vi "GETRequest.vi"(6 "Query parameters":cluster{"key":string, "value":string}[](array[cluster]), 8 "error in (no error)":errorcluster, 9 "Parameter":string, 10 "Request":string, 11 "ByteRESTBase in":refnum<class "RESTBase.lvclass">) -> (0 "error out":errorcluster, 1 "Headers":string, 2 "Body":string, 3 "ByteRESTBase out":refnum<class "RESTBase.lvclass">)   [LabVIEW 2019, in "ByteREST.lvlib" / "RESTBase.lvclass"]
doc: "Effettua una richiesta di GET al server come:\nSERVER/api/bytegs/RICHIESTA/PARAMETRO(opzionale)"
uses:
  RESTBase.lvclass
  Status_Code.ctl
  RESTBase.lvclass/RESTBase.ctl
  <vilib>/httpClient/LabVIEWHTTPClient.lvlib
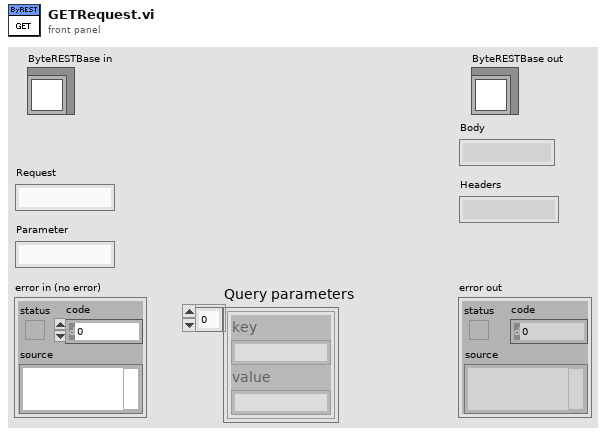
[diagram p1: front panel]
types:
  T1 = typedef "ByteREST.lvlib/RESTBase.lvclass/Status_Code.ctl" = u16
  T2 = typedef "LabVIEWHTTPClient.lvlib/ClientHandle.ctl" = refnum<k1>
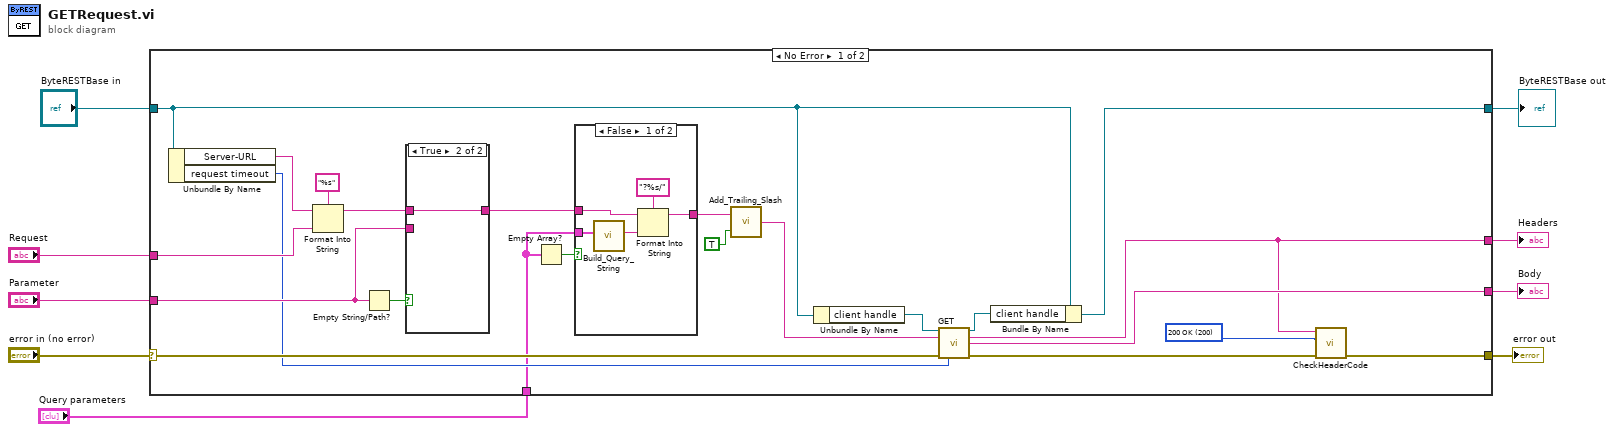
[diagram p0: block diagram]
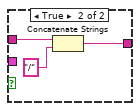
[diagram p2: hidden frame]
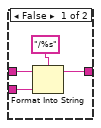
[diagram p3: hidden frame]
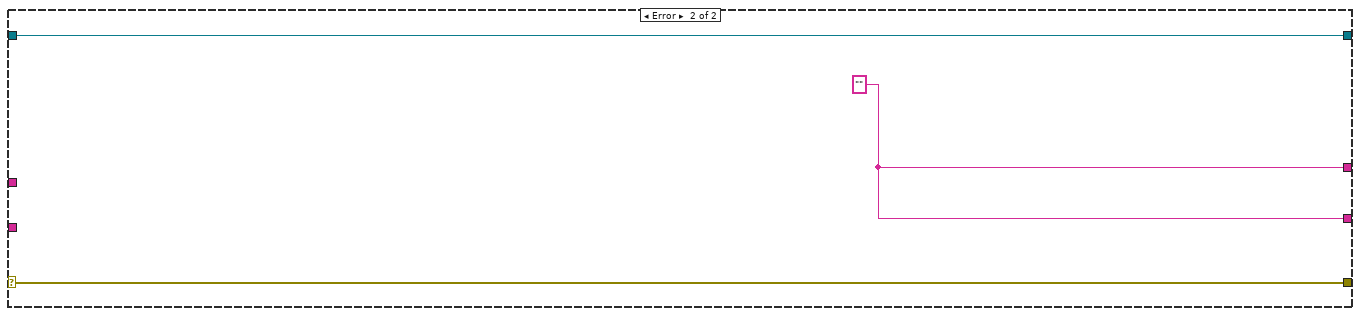
[diagram p4: hidden frame]
diagram:
  n1 = case shown="No Error" "error in (no error)" {
    selector: "error in (no error)" -> [w28 w48]
    tunnel: [w17 w48] -> w8
    tunnel: [w26 w47] -> w2
    tunnel: "ByteRESTBase in" -> [w23 w47]
    tunnel: "Request" -> [w21 _]
    tunnel: "Parameter" -> [w29 _]
    tunnel: [w25 w46] -> w5
    tunnel: [w18 w46] -> w4
    tunnel: "Query parameters" -> [w14 _]
    frame No Error {
      w19 = T1 200 items=["200 OK"=200, "201 Created"=201, "400 Bad Request"=400, "401 Unauthorized"=401, "403 Forbidden"=403, "404 Not Found"=404, "405 Method Not Allowed"=405, "406 Not Acceptable"=406, "500 Internal Server Error"=500] ("Code")
      n2 = Unbundle By Name(w23) -> ("Server-URL"=w22:string, "request timeout"=w16:i32)
      n3 = Format Into String(format string="%s" ("url"), initial string=w22, w21) -> (resulting string=w31:string)  [unwired: 1 in, 1 out]
      n4 = Empty String/Path?(string/path=w29) -> (empty?=w30:bool)
      n5 = case shown="True" w30 {
        tunnel: w31 -> [w43 w45]
        tunnel: [w41 w45] -> w13
        tunnel: w29 -> [w42 _]
        frame False {
          n6 = Format Into String(format string="/%s" ("url"), initial string=w43, w42) -> (resulting string=w41:string)  [unwired: 1 in, 1 out]
        }
        frame True {
        }
      }
      n7 = Empty Array?(array=w14) -> (empty?=w15:bool)
      n8 = case shown="False" w15 {
        tunnel: w13 -> [w36 w40]
        tunnel: [w35 w39] -> w12
        tunnel: w14 -> [w34 _]
        frame False {
          n9 = call "Build_Query_String.vi"("Query parameters"=w34) -> ("Query encoded string"=w33:string)  [unwired: 10 in]
          n10 = Format Into String(format string="?%s/" ("url"), initial string=w36, w33) -> (resulting string=w35:string)  [unwired: 1 in, 1 out]
        }
        frame True {
          n11 = Concatenate Strings(w40, "/" ("string")) -> (w39:string)
        }
      }
      n12 = call "Add_Trailing_Slash.vi"("Wanted? (True)"=TRUE, "path"=w12) -> ("path with trailing slash"=w11:string)
      n13 = Unbundle By Name(w23) -> ("client handle"=w27:T2)
      n14 = call <vilib>:"GET.vi"("client handle"=w27, "url"=w11, "error in (no error)"=w28, "timeout (10000)"=w16) -> ("client handle out"=w24:T2, "headers"=w18:string, "body"=w25:string, "error out"=w20:errorcluster)  [unwired: 8 in]
      n15 = Bundle By Name(cluster=w23, "client handle"=w24) -> (w26:refnum<class "RESTBase.lvclass">)
      n16 = call "CheckHeaderCode.vi"("error in (no error)"=w20, "Expected code (200)"=w19, "Headers"=w18) -> ("error out"=w17:errorcluster)  [unwired: 8 in]
    }
    frame Error {
      w46 = "" ("body")
    }
  }
  "error out" <- w8
  "Body" <- w5
  "Headers" <- w4
  "ByteRESTBase out" <- w2
